vi "Create From Variant.vi"(8 "error in (no error)":errorcluster, 10 "Variant":variant, 11 "JSON Array in":refnum<class "JSON Array.lvclass">) -> (0 "error out":errorcluster, 3 "JSON Array out":refnum<class "JSON Array.lvclass">)   [LabVIEW 2017, in "LVJSON.lvlib" / "JSON Array.lvclass"]
uses:
  JSON Array.lvclass
  JSON Datatype/JSON Datatype.lvclass
  JSON Array.lvclass/JSON Array.ctl
  JSON Object/JSON Object.lvclass
  C:/Users/tblair/Documents/Git Projects/LVJSON/Source/JSON Data Classes/JSON Datatype/JSON Datatype.lvclass
  JSON Numeric/JSON Numeric.lvclass
  JSON String/JSON String.lvclass
  JSON Boolean/JSON Boolean.lvclass
  JSON Numeric/New JSON Numeric.vi
  JSON String/New JSON String.vi
  JSON Boolean/New JSON Boolean.vi
  <vilib>/Utility/Data Type/NI_Data Type.lvlib
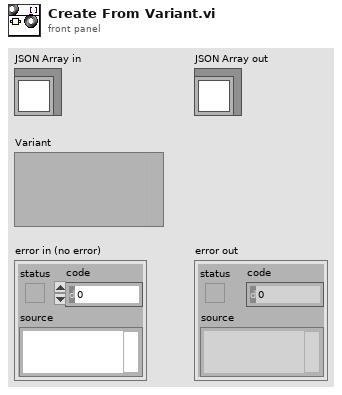
[diagram p1: front panel]
types:
  T1 = typedef "NI_Data Type.lvlib/Data Type.ctl" = enum8{"Invalid Type", "Void", "I8", "I16", "I32", "I64", "U8", "U16", "U32", "U64", "Single Float", "Double Float", "Extended Float", "Single Complex", "Double Complex", "Extended Complex", "Enum U8", "Enum U16", "Enum U32", "Enum U64", "Single Float With Unit", "Double Float With Unit", "Extended Float With Unit", "Single Complex with Unit", "Double Complex with Unit", "Extended Complex with Unit", "Boolean", "String", "Path", "Picture", "Tag", "Array", "Cluster", "Variant", "LV Variant", "Waveform", "Timestamp", "Digital Waveform", "Digital Data", "ExpressData", "Refnum", "External Data", "VI", "Poly VI", "LabVIEW Class Instance", "Fixed Point"}
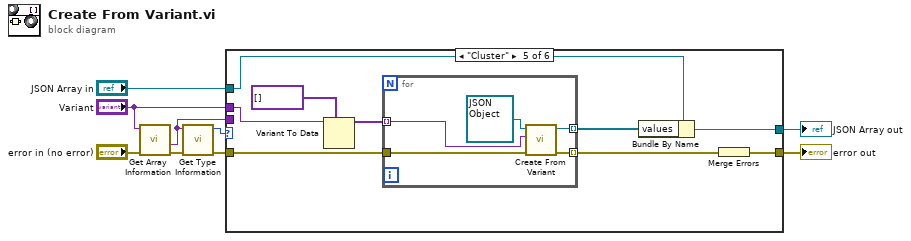
[diagram p0: block diagram]
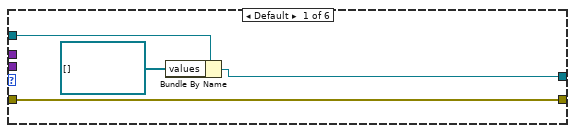
[diagram p2: hidden frame]
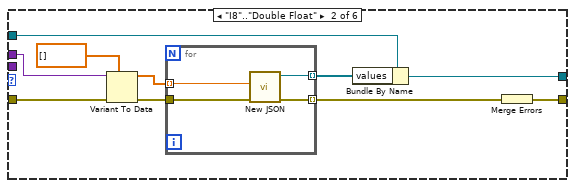
[diagram p3: hidden frame]
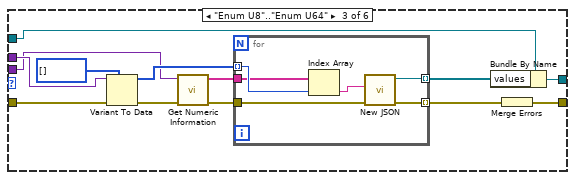
[diagram p4: hidden frame]
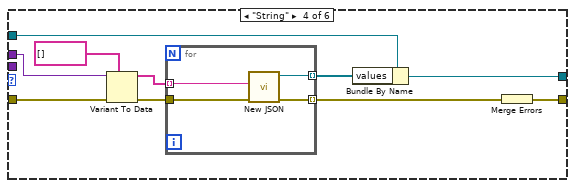
[diagram p5: hidden frame]
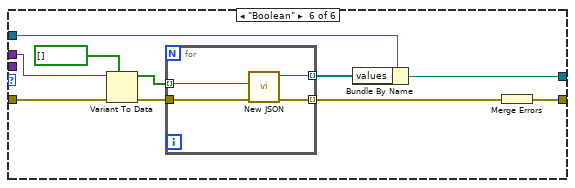
[diagram p6: hidden frame]
diagram:
  n1 = call <vilib>:"Get Array Information.vi"("error in (no error)"="error in (no error)", "Variant"="Variant") -> ("error out"=w8:errorcluster, "Array Element Data Type"=w6:variant)  [unwired: 6 in, 2 out]
  n2 = call <vilib>:"Get Type Information.vi"("error in (no error)"=w8, "Variant"=w6) -> ("error out"=w7:errorcluster, "Type"=w9:T1)  [unwired: 5 in, 3 out]
  n3 = case shown="\"Cluster\"" w9 {
    tunnel: "Variant" -> [_ w22 w39 w55 w66 w83]
    tunnel: [w11 w17 w28 w48 w67 w80] -> w3
    tunnel: w7 -> [w13 w21 w40 w54 w62 w82]
    tunnel: [w13 w14 w31 w52 w69 w75] -> w2
    tunnel: w6 -> [_ _ w34 _ _ _]
    tunnel: "JSON Array in" -> [w12 w19 w30 w50 w68 w81]
    frame Default {
      n4 = Bundle By Name(cluster=w12, "values"=refnum<class "JSON Datatype.lvclass">[] []) -> (w11:refnum<class "JSON Array.lvclass">)
    }
    frame "I8".."Double Float" {
      n5 = Variant To Data(error in=w21, type=dbl[] [], Variant=w22) -> (data=w20:dbl[], error out=w15:errorcluster)
      n6 = for {
        tunnel: w20 -> [w27] mode=indexing
        tunnel: [w26] -> w18 mode=indexing
        tunnel: w15 -> [w25]
        tunnel: [w24] -> w16 mode=indexing
        n7 = call-poly "New JSON.vi"("error in (no error)"=w25, "value"=w27) -> ("error out"=w24:errorcluster, "JSON String out"=w26:refnum<class "JSON Numeric.lvclass">)  [unwired: 8 in]
      }
      n8 = Bundle By Name(cluster=w19, "values"=w18) -> (w17:refnum<class "JSON Array.lvclass">)
      n9 = Merge Errors(w16) -> (w14:errorcluster)
    }
    frame "Enum U8".."Enum U64" {
      n10 = Variant To Data(error in=w40, type=u64[] [], Variant=w39) -> (data=w36:u64[], error out=w35:errorcluster)
      n11 = call <vilib>:"Get Numeric Information.vi"("error in (no error)"=w35, "Variant"=w34) -> ("error out"=w33:errorcluster, "Enum Names"=w37:string[])  [unwired: 6 in, 2 out]
      n12 = for {
        tunnel: w37 -> [w45]
        tunnel: w36 -> [w46] mode=indexing
        tunnel: [w43] -> w29 mode=indexing
        tunnel: w33 -> [w42]
        tunnel: [w41] -> w32 mode=indexing
        n13 = Index Array(array=w45, index=w46) -> (element=w44:string)
        n14 = call-poly "New JSON.vi"("error in (no error)"=w42, "value"=w44) -> ("error out"=w41:errorcluster, "JSON String out"=w43:refnum<class "JSON String.lvclass">)  [unwired: 8 in]
      }
      n15 = Bundle By Name(cluster=w30, "values"=w29) -> (w28:refnum<class "JSON Array.lvclass">)
      n16 = Merge Errors(w32) -> (w31:errorcluster)
    }
    frame "String" {
      n17 = Variant To Data(error in=w54, type=string[] [], Variant=w55) -> (data=w47:string[], error out=w53:errorcluster)
      n18 = for {
        tunnel: w47 -> [w60] mode=indexing
        tunnel: [w59] -> w49 mode=indexing
        tunnel: w53 -> [w58]
        tunnel: [w57] -> w51 mode=indexing
        n19 = call-poly "New JSON.vi"("error in (no error)"=w58, "value"=w60) -> ("error out"=w57:errorcluster, "JSON String out"=w59:refnum<class "JSON String.lvclass">)  [unwired: 8 in]
      }
      n20 = Bundle By Name(cluster=w50, "values"=w49) -> (w48:refnum<class "JSON Array.lvclass">)
      n21 = Merge Errors(w51) -> (w52:errorcluster)
    }
    frame "Cluster" {
      n22 = Variant To Data(type=variant[] [], Variant=w66) -> (data=w64:variant[])  [unwired: 1 in, 1 out]
      n23 = for {
        tunnel: w64 -> [w73] mode=indexing
        tunnel: [w72] -> w63 mode=indexing
        tunnel: w62 -> [w71]
        tunnel: [w70] -> w61 mode=indexing
        n24 = call-dynamic "Create From Variant.vi"("error in (no error)"=w71, "Variant"=w73, "JSON Object in"=refnum<class "JSON Object.lvclass"> refnum ("JSON Array in")) -> ("error out"=w70:errorcluster, "JSON Object out"=w72:refnum<class "JSON Object.lvclass">)  [unwired: 7 in]
      }
      n25 = Bundle By Name(cluster=w68, "values"=w63) -> (w67:refnum<class "JSON Array.lvclass">)
      n26 = Merge Errors(w61) -> (w69:errorcluster)
    }
    frame "Boolean" {
      n27 = Variant To Data(error in=w82, type=bool[] [], Variant=w83) -> (data=w79:bool[], error out=w77:errorcluster)
      n28 = for {
        tunnel: w79 -> [w88] mode=indexing
        tunnel: [w87] -> w78 mode=indexing
        tunnel: w77 -> [w86]
        tunnel: [w85] -> w76 mode=indexing
        n29 = call-poly "New JSON.vi"("error in (no error)"=w86, "value"=w88) -> ("error out"=w85:errorcluster, "JSON String out"=w87:refnum<class "JSON Boolean.lvclass">)  [unwired: 8 in]
      }
      n30 = Bundle By Name(cluster=w81, "values"=w78) -> (w80:refnum<class "JSON Array.lvclass">)
      n31 = Merge Errors(w76) -> (w75:errorcluster)
    }
  }
  "error out" <- w2
  "JSON Array out" <- w3
